vi "Teleop.vi"(10 "Match Info":T1={"Autonomous Elapsed Seconds"=0.0, "TeleOp Elapsed Seconds"=0.0, "Disabled Elapsed Seconds"=0.0, "Visited Autonomous"=FALSE, "Visited TeleOp"=FALSE, "Visited Disabled"=FALSE, "Autonomous Settings"={"Autonomous Style"=enum."Independent", "VI Refnum"=refnum}}, 11 "Call Context":T2) -> ()   [LabVIEW 2016]
doc: "This VI is called for each TeleOp packet received from the DS where the robot is not disabled. It is often used to read from the joysticks and update I/O or to update setpoints for timed control loops. It should complete and return within 20 milliseconds or it may miss DS packets."
uses:
  <vilib>/Rock Robotics/WPI/DriverStation/WPI_DriverStationDerivedRobotMode.ctl
  <vilib>/Rock Robotics/WPI/DriverStation/WPI_DriverStationMatch Info.ctl
  <vilib>/Rock Robotics/WPI/Solenoid/WPI_SolenoidValue.ctl
  <vilib>/Rock Robotics/WPI/Ultrasonic/WPI_UltrasonicRangeUnits.ctl
  <vilib>/Rock Robotics/WPI/Utilities/WPI_GetSetVariantRefNum.vi
  <vilib>/Rock Robotics/Network Tables/NT Write Boolean Array.vi
  <vilib>/Rock Robotics/Network Tables/NT Write Numeric Array.vi
  <vilib>/Rock Robotics/Network Tables/NT Read Boolean.vi
  <vilib>/Rock Robotics/Network Tables/NT Read Number.vi
  <vilib>/Rock Robotics/WPI/Ultrasonic/WPI_SonarSRF04DigitalRefNum Registry Get.vi
  <vilib>/Rock Robotics/WPI/Ultrasonic/WPI_SonarSRF04DigitalGetRange.vi
  Robot Global Data.vi
  <vilib>/Rock Robotics/WPI/Solenoid/WPI_SolenoidSetEnum.vi
panel:
  in  "reset angle":bool
  out "shifter toggle":dbl
  out "Angle":dbl
  out "dis":dbl
  out "Numeric 2":dbl
  out "Numeric":dbl
  in  "invert?":bool
  in  "intput":bool
  out "Sample Slider 0":dbl(slide) scale=0.0..5.0
  out "Sample Boolean 1":bool
  out "Sample Boolean 0":bool
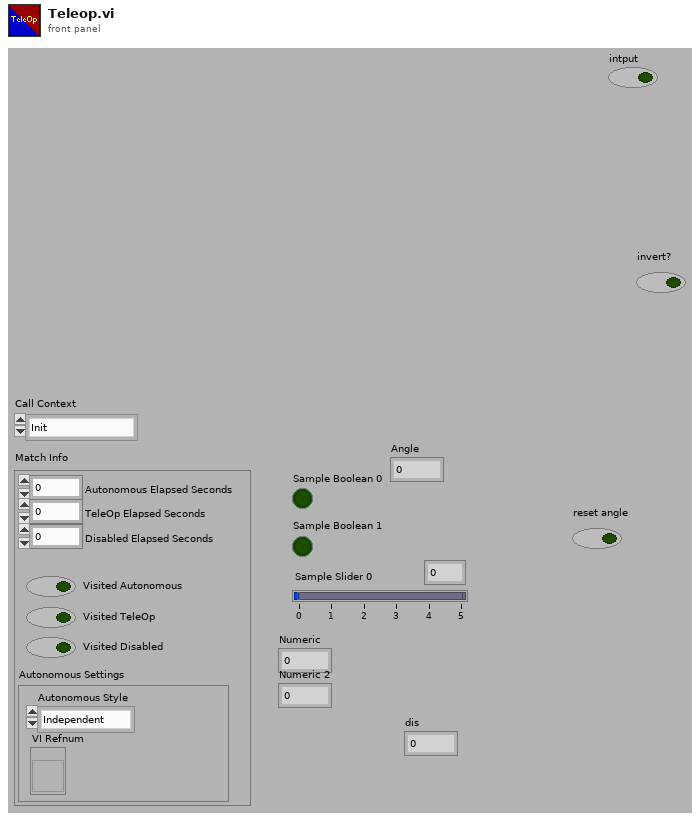
[diagram p1: front panel]
types:
  T1 = typedef "WPI_DriverStationMatch Info.ctl" = cluster{"Autonomous Elapsed Seconds":dbl, "TeleOp Elapsed Seconds":dbl, "Disabled Elapsed Seconds":dbl, "Visited Autonomous":bool, "Visited TeleOp":bool, "Visited Disabled":bool, "Autonomous Settings":cluster{"Autonomous Style":enum16{"Iterative", "Independent"}, "VI Refnum":refnum<vi>}}
  T2 = typedef "WPI_DriverStationDerivedRobotMode.ctl" = enum16{"Init", "Execute", "Stop"}
  T3 = typedef "WPI_SolenoidValue.ctl" = enum16{"Off", "On", "Forward", "Reverse"}
  T4 = typedef "WPI_UltrasonicRangeUnits.ctl" = enum16{"inches", "mm"}
  T5 = typedef "WPI_JoystickDevRef.ctl" = cluster{"Device":T6}
  T6 = typedef "WPI_JoystickDeviceEnum.ctl" = enum16{"USB 0", "USB 1", "USB 2", "USB 3", "USB 4", "USB 5"}
  T7 = typedef "WPI_RobotDriveDevRef.ctl" = cluster{"DevStatus":errorcluster, "Motors[]":T8[], "Square Inputs":bool, "Max Output":dbl}
  T8 = typedef "WPI_MotorControlDeviceRef.ctl" = cluster{"DeviceStatus":errorcluster, "Type":T9, "PWM":cluster{"PWM Channel":T10, "DeadBand":T11}, "CAN":cluster{"Device Number":u8, "SetOutput VI Ref":variant, "GetOutput VI Ref":variant, "Enable VI Ref":variant, "Disable VI Ref":variant, "Data":variant}, "Invert":bool}
  T9 = typedef "WPI_MotorControlType.ctl" = enum16{"PWM", "CAN"}
  T10 = typedef "FPGA_DIOPWMChannel.ctl" = enum8{"PWM 0", "PWM 1", "PWM 2", "PWM 3", "PWM 4", "PWM 5", "PWM 6", "PWM 7", "PWM 8", "PWM 9", "PWM MXP 0", "PWM MXP 1", "PWM MXP 2", "PWM MXP 3", "PWM MXP 4", "PWM MXP 5", "PWM MXP 6", "PWM MXP 7", "PWM MXP 8", "PWM MXP 9", "Invalid"}
  T11 = typedef "WPI_PWMDeadband.ctl" = cluster{"Name":string, "maxPositivePwm":i32, "minPositivePwm":i32, "centerPwm":i32, "maxNegativePwm":i32, "minNegativePwm":i32, "angularRange":u16}
  T12 = typedef "WPI_SolenoidDevRef.ctl" = cluster{"DevStatus":errorcluster, "Pneumatics Control Module":u8, "Forward Solenoid Channel":T13, "Reverse Solenoid Channel":T13}
  T13 = typedef "WPI_SolenoidChannel.ctl" = enum8{"Solenoid 0", "Solenoid 1", "Solenoid 2", "Solenoid 3", "Solenoid 4", "Solenoid 5", "Solenoid 6", "Solenoid 7", "Invalid"}
  T14 = typedef "WPI_GyroDevRef.ctl" = cluster{"DevStatus":errorcluster, "Analog Channel":T15, "Offset":dbl, "Gain (VoltsPerDegree/Second)":dbl, "Gyro Type":enum16{"Analog", "XRS450"}, "Handle":i32, "SPI Bus":T16, "Device Found":bool, "Sample Rate":dbl, "Calibrate On Open":bool}
  T15 = typedef "FPGA_AIChannel.ctl" = enum8{"AI 0", "AI 1", "AI 2", "AI 3", "AI MXP 0", "AI MXP 1", "AI MXP 2", "AI MXP 3", "Invalid"}
  T16 = typedef "spi_bus.ctl" = enum16{"SPI On-Board, CS0", "SPI On-Board, CS1", "SPI On-Board, CS2", "SPI On-Board, CS3", "SPI MXP", "Invalid"}
  T17 = typedef "WPI_UltrasonicDeviceRef.ctl" = cluster{"DevStatus":errorcluster, "Ping Channel":T18, "Echo Channel":T18, "CntIndex":T19}
  T18 = typedef "FPGA_DIOChannel.ctl" = enum8{"DIO 0", "DIO 1", "DIO 2", "DIO 3", "DIO 4", "DIO 5", "DIO 6", "DIO 7", "DIO 8", "DIO 9", "DIO MXP 0", "DIO MXP 1", "DIO MXP 2", "DIO MXP 3", "DIO MXP 4", "DIO MXP 5", "DIO MXP 6", "DIO MXP 7", "DIO MXP 8", "DIO MXP 9", "DIO MXP 10", "DIO MXP 11", "DIO MXP 12", "DIO MXP 13", "DIO MXP 14", "DIO MXP 15", "SPI Port CS1", "SPI Port CS2", "SPI Port CS3", "SPI Port MISO", "SPI Port MOSI", "Invalid"}
  T19 = typedef "FPGA_CounterCtrSystemIndex.ctl" = enum8{"Ctr 0", "Ctr 1", "Ctr 2", "Ctr 3", "Ctr 4", "Ctr 5", "Ctr 6", "Ctr 7", "Invalid"}
  T20 = typedef "WPI_EncoderDevRef.ctl" = cluster{"DevStatus":errorcluster, "EncoderIndex":T21, "CounterIndex":T19, "DistancePerCount":dbl, "Decoding Type":T22}
  T21 = typedef "FPGA_EncoderIdx.ctl" = enum8{"Enc 0", "Enc 1", "Enc 2", "Enc 3", "Enc 4", "Enc 5", "Enc 6", "Enc 7", "Invalid"}
  T22 = typedef "WPI_EncoderType.ctl" = enum16{"1x", "2x", "4x"}
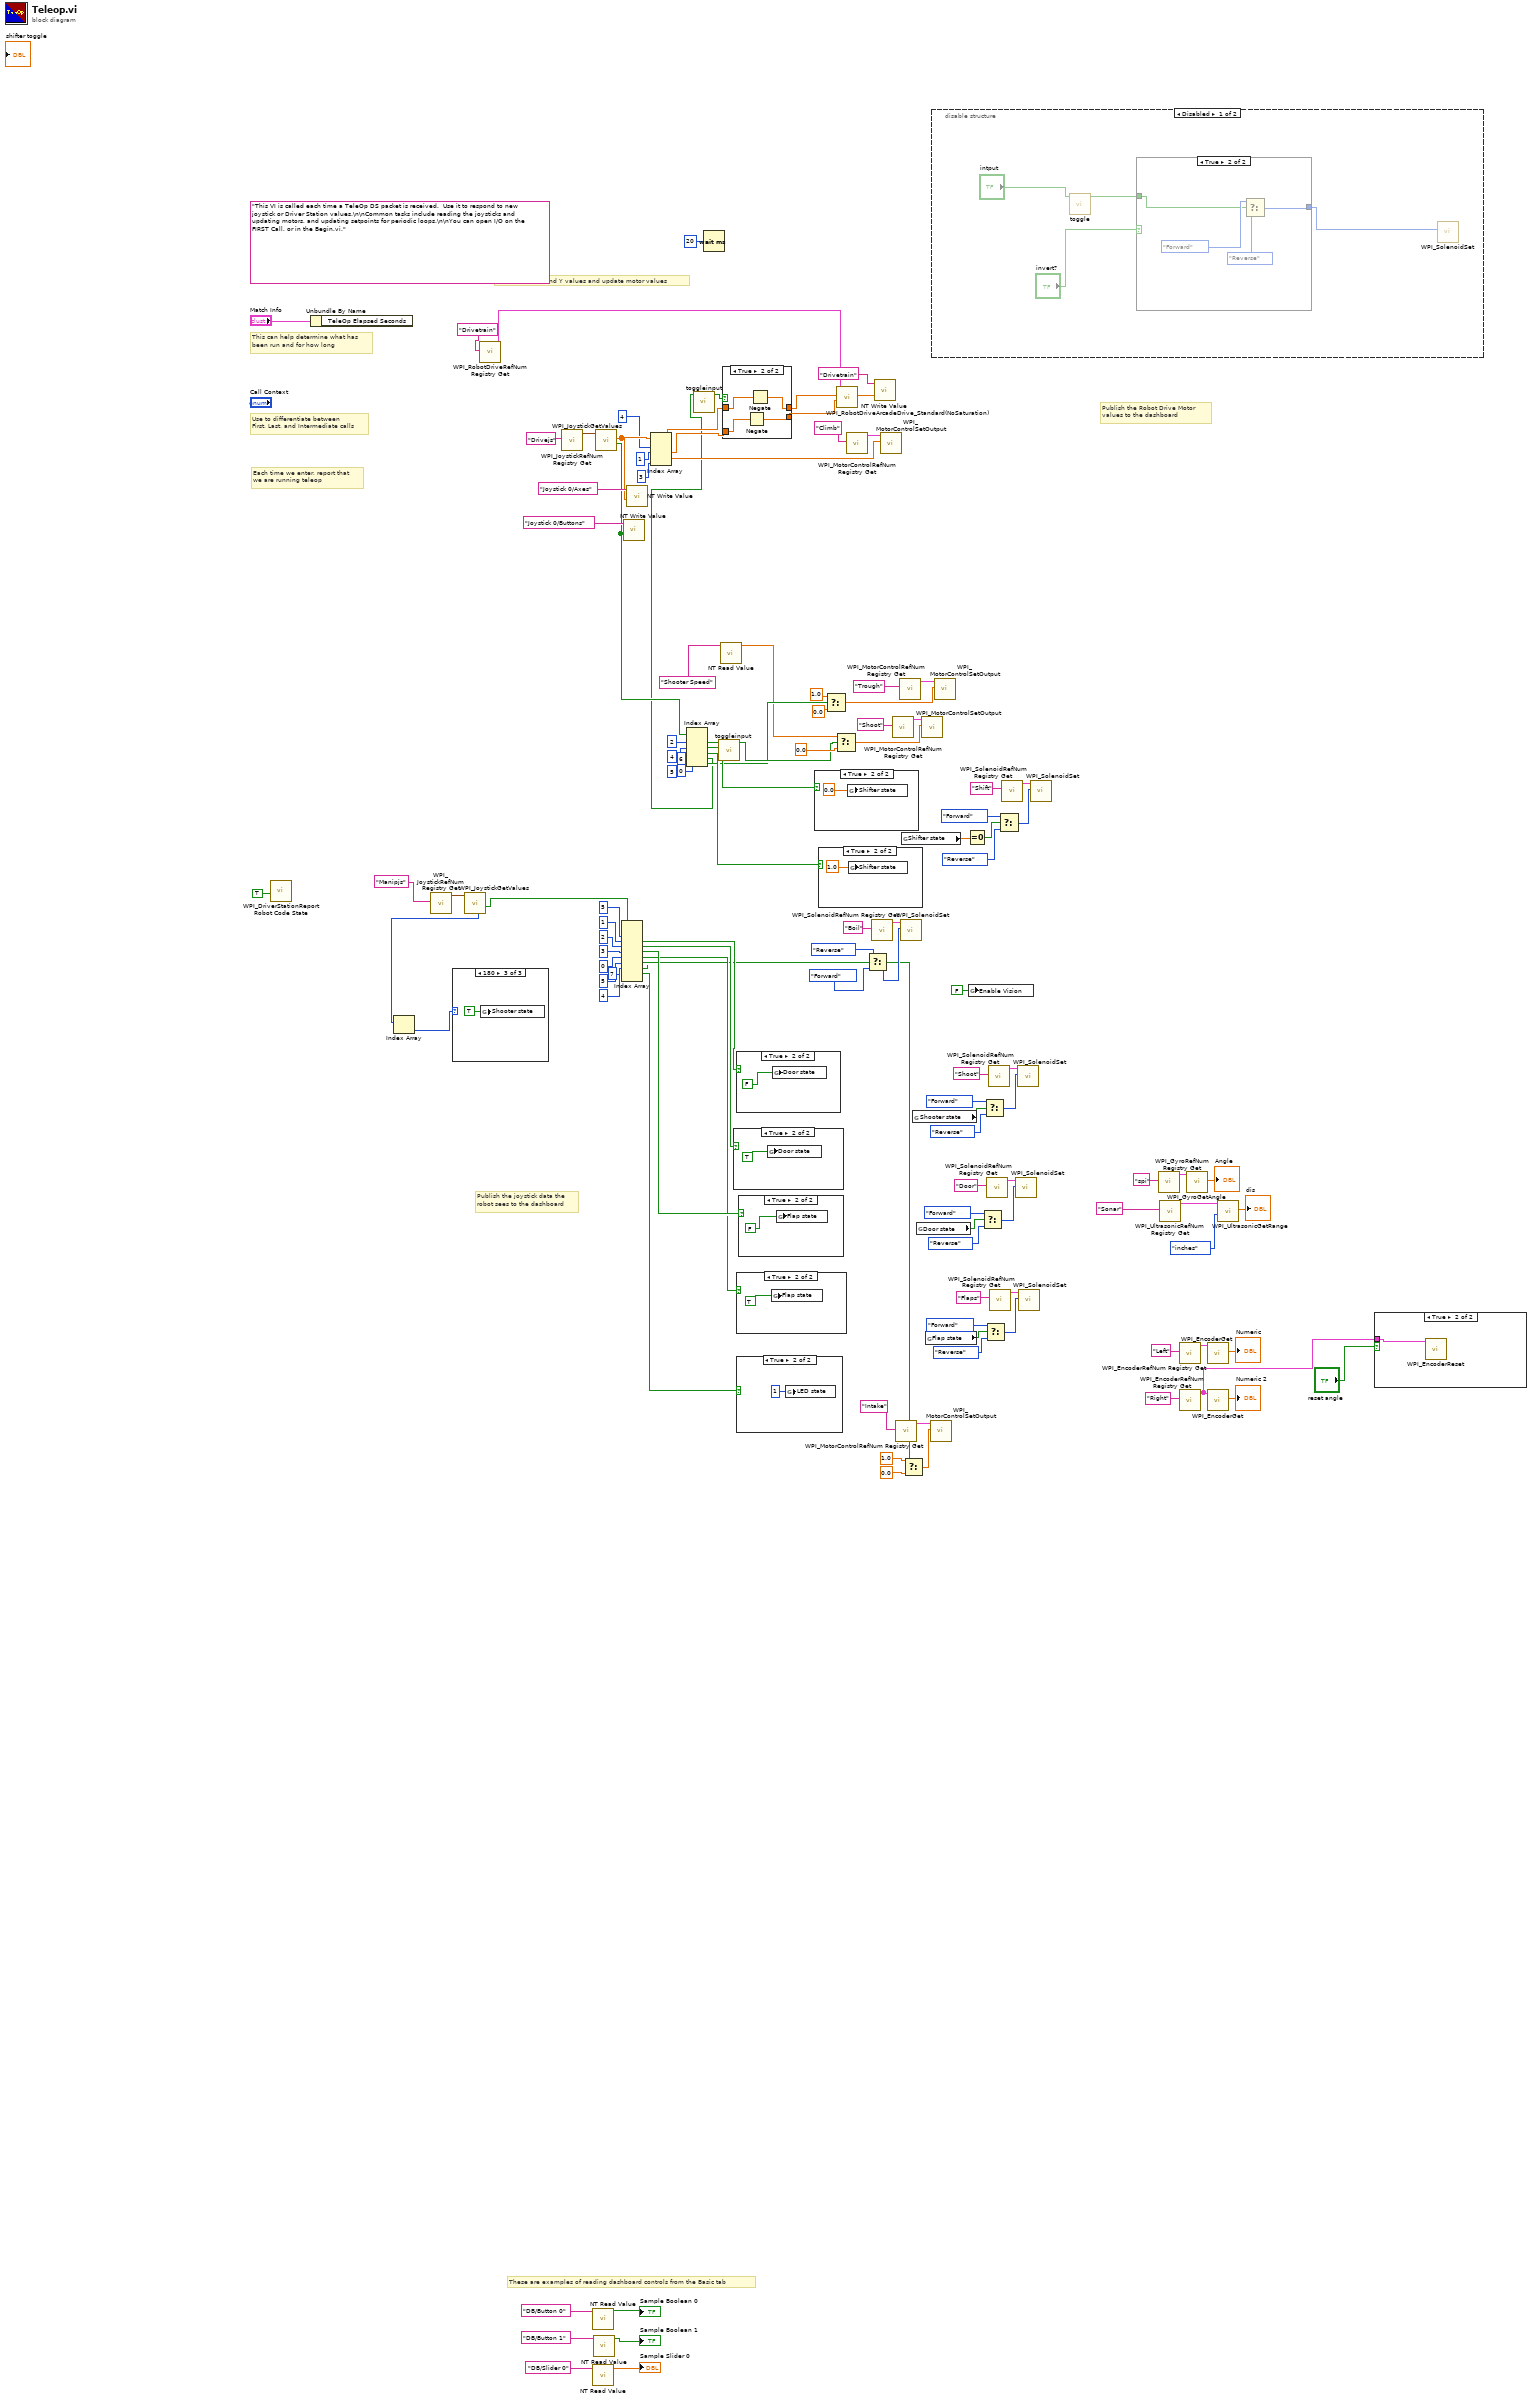
[diagram p0: block diagram]
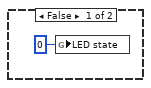
[diagram p3: hidden frame]
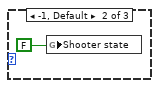
[diagram p5: hidden frame]
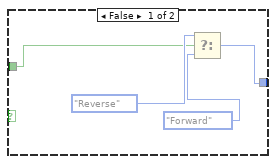
[diagram p13: hidden frame]
diagram:
  (unwired) "This VI is called each time a TeleOp DS packet is received.  Use it to respond to new joystick or Driver Station values.\n\nCommon tasks include reading the joysticks and updating motors, and updating setpoints for periodic loops.\n\nYou can open I/O on the FIRST Call, or in the Begin.vi."
  # "These are examples of reading dashboard controls from the Basic tab"
  # "Publish the Robot Drive Motor\nvalues to the dashboard"
  # "Publish the joystick data the\nrobot sees to the dashboard"
  # "Each time we enter, report that\nwe are running teleop"
  # "Use to differentiate between\nFirst, Last, and Intermediate calls"
  # "This can help determine what has\nbeen run and for how long"
  # "Read Joystick X and Y values and update motor values"
  n1 = call <vilib>:"WPI_DriverStationReport Robot Code State.vi"("TeleOp"=TRUE ("Autonomous")) -> ()  [unwired: 10 in, 1 out]
  n2 = Unbundle By Name("Match Info") -> ()  [unwired: 1 out]
  n3 = call <vilib>:"WPI_JoystickRefNum Registry Get.vi"("refnum name"="Manipjs") -> ("JoystickDevRef"=w75:T5)  [unwired: 1 in, 9 out]
  n4 = call <vilib>:"WPI_JoystickGetValues.vi"("JoystickDevRef"=w75) -> ("Buttons"=w74:bool[], "POVs"=w16:i16[])  [unwired: 6 in, 3 out]
  n5 = Index Array(array=w16) -> (element=w15:i16)  [unwired: 1 in]
  n6 = case shown="180" w15 {
    frame 0 {
    }
    frame -1, Default {
      n7 = global write "Robot Global Data.vi" "Shooter state"(FALSE ("Door state")) -> ()
    }
    frame 180 {
      n8 = global write "Robot Global Data.vi" "Shooter state"(TRUE ("Shooter state")) -> ()
    }
  }
  n9 = call <vilib>:"WPI_RobotDriveRefNum Registry Get.vi"("refnum name"="Drivetrain") -> ("RobotDriveDevRef"=w120:T7)  [unwired: 1 in, 9 out]
  n10 = call <vilib>:"WPI_JoystickRefNum Registry Get.vi"("refnum name"="Drivejs") -> ("JoystickDevRef"=w118:T5)  [unwired: 1 in, 9 out]
  n11 = call-poly <vilib>:"NT Read Value.vi"("Name"="DB/Button 0" ("refnum name")) -> ("Boolean"=→"Sample Boolean 0":bool)  [unwired: 9 in, 1 out]
  n12 = call-poly <vilib>:"NT Read Value.vi"("Name"="DB/Slider 0" ("refnum name")) -> ("Numeric"=→"Sample Slider 0":dbl)  [unwired: 9 in, 1 out]
  n13 = call-poly <vilib>:"NT Read Value.vi"("Name"="DB/Button 1" ("refnum name")) -> ("Boolean"=→"Sample Boolean 1":bool)  [unwired: 9 in, 1 out]
  n14 = call <vilib>:"WPI_JoystickGetValues.vi"("JoystickDevRef"=w118) -> ("Buttons"=w73:bool[], "Axes"=w114:dbl[])  [unwired: 6 in, 3 out]
  n15 = Index Array(array=w74, index #1=5 ("index"), index #2=1 ("index"), index #3=2 ("index"), index #4=3 ("index"), index #5=0 ("index"), index #6=5 ("index"), index #7=4 ("index"), index #8=7 ("index")) -> (element #2=w39:bool, element #3=w38:bool, element #4=w35:bool, element #5=w33:bool, element #6=w24:bool, element #7=w17:bool, element #8=w4:bool)  [unwired: 1 in, 2 out]
  n16 = call-poly <vilib>:"NT Write Value.vi"("Boolean Array"=w73, "Name"="Joystick 0/Buttons") -> ()  [unwired: 9 in, 1 out]
  n17 = call-poly <vilib>:"NT Write Value.vi"("Numeric Array"=w114, "Name"="Joystick 0/Axes") -> ()  [unwired: 9 in, 1 out]
  n18 = Index Array(array=w114, index #1=4 ("index"), index #2=1 ("index"), index #4=3 ("index")) -> (element #1=w30:dbl, element #2=w28:dbl, element #3=w22:dbl)  [unwired: 1 in, 1 out]
  n19 = Index Array(array=w73, index #1=2 ("index"), index #2=4 ("index"), index #3=5 ("index"), index #4=6 ("index"), index #5=0 ("index")) -> (element #1=w68:bool, element #2=w43:bool, element #3=w42:bool, element #4=w12:bool, element #5=w19:bool)
  n20 = call "toggleinput.vi"("Boolean"=w12) -> ("Boolean 2"=w26:bool)  [unwired: 10 in]
  n21 = Wait (ms)(milliseconds to wait=u32 20) -> ()  [unwired: 1 out]
  n22 = call "toggleinput.vi"("Boolean"=w68) -> ("Boolean 2"=w61:bool)  [unwired: 10 in]
  n23 = call-poly <vilib>:"NT Read Value.vi"("Name"="Shooter Speed") -> ("Numeric"=w13:dbl)  [unwired: 9 in, 1 out]
  n24 = case shown="True" w26 {
    tunnel: w30 -> [w126 w130]
    tunnel: [w126 w129] -> w29
    tunnel: w28 -> [w125 w128]
    tunnel: [w125 w127] -> w27
    frame False {
    }
    frame True {
      n25 = Negate(x=w128) -> (-x=w127:dbl)
      n26 = Negate(x=w130) -> (-x=w129:dbl)
    }
  }
  n27 = case shown="True" w38 {
    frame False {
    }
    frame True {
      n28 = global write "Robot Global Data.vi" "Door state"(TRUE ("Door state")) -> ()
    }
  }
  n29 = case shown="True" w39 {
    frame False {
    }
    frame True {
      n30 = global write "Robot Global Data.vi" "Door state"(FALSE ("Door state")) -> ()
    }
  }
  n31 = case shown="True" w33 {
    frame False {
    }
    frame True {
      n32 = global write "Robot Global Data.vi" "Flap state"(TRUE ("Door state")) -> ()
    }
  }
  n33 = case shown="True" w4 {
    frame False {
      n34 = global write "Robot Global Data.vi" "LED state"(i8 0 ("LED state")) -> ()
    }
    frame True {
      n35 = global write "Robot Global Data.vi" "LED state"(i8 1 ("LED state")) -> ()
    }
  }
  n36 = case shown="True" w35 {
    frame False {
    }
    frame True {
      n37 = global write "Robot Global Data.vi" "Flap state"(FALSE ("Door state")) -> ()
    }
  }
  n38 = case shown="True" w43 {
    frame False {
    }
    frame True {
      n39 = global write "Robot Global Data.vi" "Shifter state"(0.0 ("shifter toggle")) -> ()
    }
  }
  n40 = case shown="True" w42 {
    frame False {
    }
    frame True {
      n41 = global write "Robot Global Data.vi" "Shifter state"(1.0 ("shifter toggle")) -> ()
    }
  }
  n42 = Select(t=1.0, s=w19, f=0.0) -> (s? t:f=w60:dbl)
  n43 = Select(t=w13, s=w61, f=0.0) -> (s? t:f=w67:dbl)
  n44 = call <vilib>:"WPI_RobotDriveArcadeDrive_Standard(NoSaturation).vi"("Y axis value"=w27, "X axis value"=w29, "RobotDriveDevRef"=w120) -> ("Motor Values"=w107:dbl[])  [unwired: 1 in, 7 out]
  n45 = call <vilib>:"WPI_MotorControlRefNum Registry Get.vi"("refnum name"="Climb") -> ("MotorControlDevRef"=w102:T8)  [unwired: 9 in, 1 out]
  n46 = Select(t=WPI_SolenoidValue."Reverse" ("Value"), s=w17, f=WPI_SolenoidValue."Forward" ("Value")) -> (s? t:f=w82:T3)
  n47 = call <vilib>:"WPI_SolenoidRefNum Registry Get.vi"("refnum name"="Boil") -> ("SolenoidDevRef"=w84:T12)  [unwired: 9 in, 1 out]
  n48 = call-poly <vilib>:"NT Write Value.vi"("Numeric Array"=w107, "Name"="Drivetrain") -> ()  [unwired: 9 in, 1 out]
  n49 = call <vilib>:"WPI_MotorControlSetOutput.vi"("Output"=w22, "MotorControlDevRef"=w102) -> ()  [unwired: 7 in, 3 out]
  n50 = call <vilib>:"WPI_MotorControlRefNum Registry Get.vi"("refnum name"="Shoot") -> ("MotorControlDevRef"=w70:T8)  [unwired: 9 in, 1 out]
  n51 = call <vilib>:"WPI_MotorControlRefNum Registry Get.vi"("refnum name"="Intake") -> ("MotorControlDevRef"=w57:T8)  [unwired: 9 in, 1 out]
  n52 = call <vilib>:"WPI_MotorControlRefNum Registry Get.vi"("refnum name"="Trough") -> ("MotorControlDevRef"=w64:T8)  [unwired: 9 in, 1 out]
  n53 = call-poly <vilib>:"WPI_SolenoidSet.vi"("Value"=w82, "SolenoidDevRef"=w84) -> ()  [unwired: 8 in, 2 out]
  n54 = global read "Robot Global Data.vi" "Shifter state"() -> (w40:dbl)
  n55 = Select(t=1.0, s=w24, f=0.0) -> (s? t:f=w56:dbl)
  n56 = global read "Robot Global Data.vi" "Shooter state"() -> (w6:bool)
  n57 = global read "Robot Global Data.vi" "Door state"() -> (w37:bool)
  n58 = call <vilib>:"WPI_MotorControlSetOutput.vi"("Output"=w67, "MotorControlDevRef"=w70) -> ()  [unwired: 7 in, 3 out]
  n59 = global read "Robot Global Data.vi" "Flap state"() -> (w32:bool)
  n60 = call <vilib>:"WPI_MotorControlSetOutput.vi"("Output"=w56, "MotorControlDevRef"=w57) -> ()  [unwired: 7 in, 3 out]
  n61 = disable-structure shown="Disabled" {
    frame Disabled {
      n62 = call "toggle.vi"("Boolean"="intput") -> ("Boolean 2"=w140:bool)  [unwired: 10 in]
      n63 = case shown="True" "invert?" {
        tunnel: [w145 w148] -> w139
        tunnel: w140 -> [w143 w147]
        frame False {
          n64 = Select(t=WPI_SolenoidValue."Reverse" ("Value"), s=w143, f=WPI_SolenoidValue."Forward" ("Value")) -> (s? t:f=w145:T3)
        }
        frame True {
          n65 = Select(t=WPI_SolenoidValue."Forward" ("Value"), s=w147, f=WPI_SolenoidValue."Reverse" ("Value")) -> (s? t:f=w148:T3)
        }
      }
      n66 = call-poly <vilib>:"WPI_SolenoidSet.vi"("Value"=w139) -> ()  [unwired: 9 in, 2 out]
    }
    frame Enabled {
    }
  }
  n67 = call <vilib>:"WPI_MotorControlSetOutput.vi"("Output"=w60, "MotorControlDevRef"=w64) -> ()  [unwired: 7 in, 3 out]
  n68 = Equal To 0?(x=w40) -> (x = 0?=w41:bool)
  n69 = global write "Robot Global Data.vi" "Enable Vision"(FALSE ("Enable Vision")) -> ()
  n70 = Select(t=WPI_SolenoidValue."Forward" ("Value"), s=w37, f=WPI_SolenoidValue."Reverse" ("Value")) -> (s? t:f=w98:T3)
  n71 = Select(t=WPI_SolenoidValue."Forward" ("Value"), s=w6, f=WPI_SolenoidValue."Reverse" ("Value")) -> (s? t:f=w8:T3)
  n72 = Select(t=WPI_SolenoidValue."Forward" ("Value"), s=w32, f=WPI_SolenoidValue."Reverse" ("Value")) -> (s? t:f=w93:T3)
  n73 = call <vilib>:"WPI_SolenoidRefNum Registry Get.vi"("refnum name"="Door") -> ("SolenoidDevRef"=w100:T12)  [unwired: 9 in, 1 out]
  n74 = call <vilib>:"WPI_SolenoidRefNum Registry Get.vi"("refnum name"="Shoot") -> ("SolenoidDevRef"=w10:T12)  [unwired: 9 in, 1 out]
  n75 = call <vilib>:"WPI_SolenoidRefNum Registry Get.vi"("refnum name"="Flaps") -> ("SolenoidDevRef"=w95:T12)  [unwired: 9 in, 1 out]
  n76 = Select(t=WPI_SolenoidValue."Forward" ("Value"), s=w41, f=WPI_SolenoidValue."Reverse" ("Value")) -> (s? t:f=w51:T3)
  n77 = call <vilib>:"WPI_SolenoidRefNum Registry Get.vi"("refnum name"="Shift") -> ("SolenoidDevRef"=w50:T12)  [unwired: 9 in, 1 out]
  n78 = call-poly <vilib>:"WPI_SolenoidSet.vi"("Value"=w98, "SolenoidDevRef"=w100) -> ()  [unwired: 8 in, 2 out]
  n79 = call-poly <vilib>:"WPI_SolenoidSet.vi"("Value"=w8, "SolenoidDevRef"=w10) -> ()  [unwired: 8 in, 2 out]
  n80 = call-poly <vilib>:"WPI_SolenoidSet.vi"("Value"=w93, "SolenoidDevRef"=w95) -> ()  [unwired: 8 in, 2 out]
  n81 = call-poly <vilib>:"WPI_SolenoidSet.vi"("Value"=w51, "SolenoidDevRef"=w50) -> ()  [unwired: 8 in, 2 out]
  n82 = call <vilib>:"WPI_GyroRefNum Registry Get.vi"("refnum name"="spi") -> ("GyroDevRef"=w2:T14)  [unwired: 9 in, 1 out]
  n83 = call-poly <vilib>:"WPI_UltrasonicRefNum Registry Get.vi"("refnum name"="Sonar") -> ("SonarSRF04DevRef"=w79:T17)  [unwired: 9 in, 1 out]
  n84 = call <vilib>:"WPI_EncoderRefNum Registry Get.vi"("refnum name"="Left") -> ("EncoderDevRef"=w88:T20)  [unwired: 9 in, 1 out]
  n85 = call <vilib>:"WPI_EncoderRefNum Registry Get.vi"("refnum name"="Right") -> ("EncoderDevRef"=w1:T20)  [unwired: 9 in, 1 out]
  n86 = call <vilib>:"WPI_GyroGetAngle.vi"("GyroDevRef"=w2) -> ("Angle"=→"Angle":dbl)  [unwired: 6 in, 4 out]
  n87 = call <vilib>:"WPI_EncoderGet.vi"("EncoderDevRef"=w88) -> ("Distance"=→"Numeric":dbl)  [unwired: 5 in, 5 out]
  n88 = call <vilib>:"WPI_EncoderGet.vi"("EncoderDevRef"=w1) -> ("Distance"=→"Numeric 2":dbl)  [unwired: 5 in, 5 out]
  n89 = call-poly <vilib>:"WPI_UltrasonicGetRange.vi"("Range Units"=WPI_UltrasonicRangeUnits."inches", "SonarSRF04DevRef"=w79) -> ("Distance"=→"dis":dbl)  [unwired: 7 in, 2 out]
  n90 = case shown="True" "reset angle" {
    tunnel: w1 -> [_ w151]
    frame False {
    }
    frame True {
      n91 = call <vilib>:"WPI_EncoderReset.vi"("EncoderDevRef"=w151) -> ()  [unwired: 9 in, 2 out]
    }
  }
